vi "parseATIcalFile.vi"(11 "Calibration File":path) -> (0 "error out":errorcluster, 2 "Calibration array":dbl[][](array[numeric]))   [LabVIEW 2022 SP3]
panel:
  out "text":string
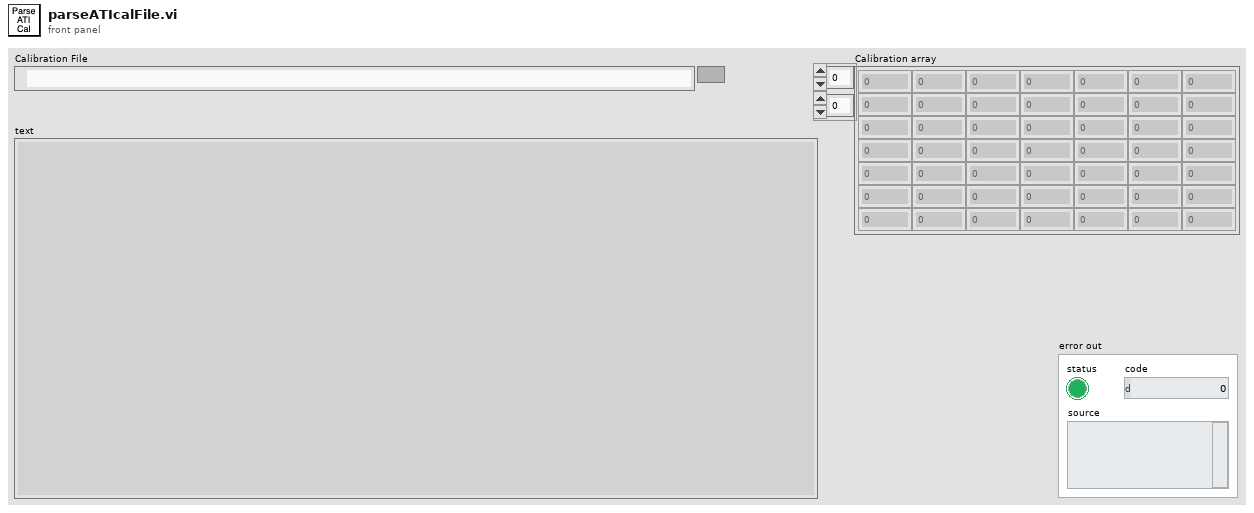
[diagram p1: front panel]
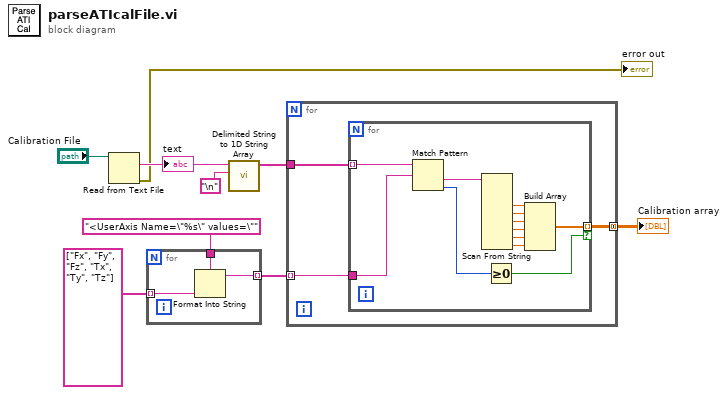
[diagram p0: block diagram]
diagram:
  n1 = Read from Text File(file (use dialog)="Calibration File") -> (text=w2:string, error out=→"error out":errorcluster)  [unwired: 3 in, 2 out]
  "text" <- w2
  n2 = for {
    tunnel: "<UserAxis Name=\"%s\" values=\"" ("text") -> [w12]
    tunnel: string[] ["Fx", "Fy", "Fz", "Tx", "Ty", "Tz"] -> [w11] mode=indexing
    tunnel: [w10] -> w4 mode=indexing
    n3 = Format Into String(format string=w12, w11) -> (resulting string=w10:string)  [unwired: 2 in, 1 out]
  }
  n4 = call <vilib>:"Delimited String to 1D String Array.vi"("delimiter"="\n", "delimited string"=w2) -> ("string array"=w5:string[])  [unwired: 9 in]
  n5 = for {
    tunnel: w5 -> [w15]
    tunnel: w4 -> [w14] mode=indexing
    tunnel: [w13] -> w3 mode=concatenating
    n6 = for {
      tunnel: w15 -> [w27] mode=indexing
      tunnel: w14 -> [w26]
      tunnel: [w16] -> w13 mode=indexing if=w24
      n7 = Match Pattern(string=w27, regular expression=w26) -> (after substring=w23:string, offset past match=w25:i32)  [unwired: 1 in, 2 out]
      n8 = Scan From String(input string=w23) -> (output 1=w22:dbl, output 2=w21:dbl, output 3=w20:dbl, output 4=w19:dbl, output 5=w18:dbl, output 6=w17:dbl)  [unwired: 9 in, 3 out]
      n9 = Greater Or Equal To 0?(x=w25) -> (x >= 0?=w24:bool)
      n10 = Build Array(w22, w21, w20, w19, w18, w17) -> (w16:dbl[])
    }
  }
  "Calibration array" <- w3
